vi "Ex 06 - B-Scan.vi"() -> ()   [LabVIEW 2026]
uses:
  <instrlib>/MicroPulse/Public/Data/Datatypes/MP - data formatting.ctl
  <instrlib>/MicroPulse/Public/Data/Datatypes/MP - amplitude reporting mode.ctl
  <instrlib>/MicroPulse/Public/Data/Datatypes/MP - averaging.ctl
  <instrlib>/MicroPulse/Public/Data/Datatypes/MP - transmit parameters.ctl
  <instrlib>/MicroPulse/Public/Data/Datatypes/MP - pulser voltage.ctl
  <instrlib>/MicroPulse/Public/Data/Datatypes/MP - pulse damping.ctl
  <instrlib>/MicroPulse/Public/Data/Datatypes/MP - test parameters.ctl
  <instrlib>/MicroPulse/Public/Data/Datatypes/MP - receive parameters.ctl
  <instrlib>/MicroPulse/Public/Data/Datatypes/MP - display gate.ctl
  <instrlib>/MicroPulse/Public/Data/Datatypes/MP - waveform type.ctl
  <instrlib>/MicroPulse/Public/Data/Datatypes/MP - analogue filter.ctl
  <instrlib>/MicroPulse/Public/Data/Datatypes/MP - frequency filter.ctl
  <instrlib>/MicroPulse/Public/Data/Datatypes/MP - digital filtering.ctl
  <instrlib>/MicroPulse/Public/Data/Datatypes/MP - high pass filter.ctl
  <instrlib>/MicroPulse/Public/Data/Datatypes/MP - low pass filter.ctl
  <instrlib>/MicroPulse/Public/Data/Datatypes/TCP config.ctl
  <instrlib>/MicroPulse/Public/Data/Datatypes/MP - multi-gate inspection.ctl
  <instrlib>/MicroPulse/Public/Data/Datatypes/MP - multigate inspection gate parameters.ctl
  <instrlib>/MicroPulse/Public/Data/Datatypes/MP - hysteresis level.ctl
  <instrlib>/MicroPulse/Public/Data/Datatypes/MP - multigate mode.ctl
  <instrlib>/MicroPulse/Public/Data/Datatypes/MP - echo gate parameters.ctl
  <instrlib>/MicroPulse/Public/Data/Datatypes/MP - echo gate mode.ctl
  <instrlib>/MicroPulse/Public/Data/Datatypes/MP - data output format.ctl
  <instrlib>/MicroPulse/Public/Data/Datatypes/MP - sample frequency.ctl
  <instrlib>/MicroPulse/Public/Data/Datatypes/MP - instrument type.ctl
  <instrlib>/MicroPulse/Public/Data/Datatypes/MP - fly scan range.ctl
  <instrlib>/MicroPulse/Public/Data/Datatypes/MP - inspection direction.ctl
  <instrlib>/MicroPulse/Public/Data/Datatypes/MP - encoder settings.ctl
  <instrlib>/MicroPulse/Public/Data/Datatypes/MP - encoder type.ctl
  <instrlib>/MicroPulse/Public/Data/Datatypes/MP - request system status.ctl
  <instrlib>/MicroPulse/Public/Data/Datatypes/MP - encoder mode.ctl
  <instrlib>/MicroPulse/Public/Data/Datatypes/MP - fly scan range (relative).ctl
  <instrlib>/MicroPulse/Public/Data/Datatypes/MP - inspection direction (relative).ctl
  <instrlib>/MicroPulse/Public/Data/Datatypes/MP - fly scan range (timed).ctl
  <instrlib>/MicroPulse/Public/Data/Datatypes/PNDT - colour map selector.ctl
  <instrlib>/MicroPulse/Examples/SubVIs/Main Program State - Enum.ctl
  <instrlib>/MicroPulse/Public/Data/Datatypes/MP - fly inspection tests.ctl
  <instrlib>/MicroPulse/Public/Helper VIs/Low Level/FGV - B-Scan Active - Action [Enum].ctl
  <vilib>/ErrorRing/Error Ring.xnode
  <instrlib>/MicroPulse/MicroPulse_Driver.lvlib
panel:
  in  "Centre Cursor":bool
  in  "Get Status":bool
  in  "Colour Map":T1
  out "B-Scan In Progress?":bool
  in  "Stop Test":bool
  out "B-Scan Chart":u16[][](graph)
  in  "Request System Status":T2 caption="[STS]"
  out "Current Position":dbl format="%#_6f mm"
  in  "Test Tab":T3(tab)
  in  "Data Formatting":T4={"Amplitude Mode"=enum."Peaks + Ascan for Multigate", "Averaging"=enum."None", "Coupling Level"=0} {"Coupling Level" max=4095 step=1}
  in  "Transmit Parameters":T7={"Pulse Voltage"=enum."50V", "Pulse Shape"={"Damping"=enum."660W", "Width"=250}} {"Pulse Shape"."Width" min=16 max=1010 step=50 format="%.0fns"}
  in  "Test Parameters":T10={"Test No."=1, "Tx Channel"=1, "Rx Channel"=1} {"Rx Channel" min=1 max=1024; "Tx Channel" min=1 max=1024}
  in  "Receive Parameters":T11={"Display Gate"={"Start"=0.0, "Length"=100.0}, "Delay"=0.0, "Waveform Type"=enum."Rectified Signal", "Gain"=50.0, "Analogue Filtering"={"Bandpass"=enum."No change", "Smoothing"=1}, "Digital Filtering"={"High Pass Filter"=enum."None", "Low Pass Filter"=enum."None"}} {"Delay" format="%#_g us"; "Display Gate"."Length" min=0.0 max=64000.0 step=1.0 format="%#_g us"; "Display Gate"."Start" min=0.0 max=64000.0 step=1.0 format="%#_g us"; "Analogue Filtering"."Smoothing" min=1 max=11 step=1; "Gain" min=-6.0 max=70.0 step=0.25 format="%.2fdB"}
  in  "Multi Gate Inspection":T19={"Gate 1"={"Start (us)"=15.0, "Length (us)"=10.0, "Threshold"=80, "Enabled?"=TRUE, "Max # Peaks"=8, "Hysteresis"=enum."6dB", "Mode"=enum."All Peaks In Gate", "Inverted?"=FALSE, "Colour "=16716306}, "Gate 2"={"Start (us)"=30.0, "Length (us)"=10.0, "Threshold"=50, "Enabled?"=TRUE, "Max # Peaks"=8, "Hysteresis"=enum."6dB", "Mode"=enum."All Peaks In Gate", "Inverted?"=FALSE, "Colour "=641024}, "Gate 3"={"Start (us)"=50.0, "Length (us)"=10.0, "Threshold"=30, "Enabled?"=TRUE, "Max # Peaks"=8, "Hysteresis"=enum."6dB", "Mode"=enum."All Peaks In Gate", "Inverted?"=FALSE, "Colour "=4532}, "Gate 4"={"Start (us)"=65.0, "Length (us)"=10.0, "Threshold"=10, "Enabled?"=TRUE, "Max # Peaks"=8, "Hysteresis"=enum."6dB", "Mode"=enum."All Peaks In Gate", "Inverted?"=FALSE, "Colour "=8978537}} {"Gate 4"."Max # Peaks" min=1 max=80 step=1; "Gate 4"."Threshold" min=10 step=10; "Gate 4"."Length (us)" min=0.0 max=96000.0 step=1.0; "Gate 4"."Start (us)" min=0.0 max=64000.0 step=1.0; "Gate 3"."Max # Peaks" min=1 max=80 step=1; "Gate 3"."Threshold" min=10 step=10; "Gate 3"."Length (us)" min=0.0 max=96000.0 step=1.0; "Gate 3"."Start (us)" min=0.0 max=64000.0 step=1.0; "Gate 2"."Max # Peaks" min=1 max=80 step=1; "Gate 2"."Threshold" min=10 step=10; "Gate 2"."Length (us)" min=0.0 max=96000.0 step=1.0; "Gate 2"."Start (us)" min=0.0 max=64000.0 step=1.0; "Gate 1"."Max # Peaks" min=1 max=80 step=1; "Gate 1"."Threshold" min=10 step=10; "Gate 1"."Length (us)" min=0.0 max=96000.0 step=1.0; "Gate 1"."Start (us)" min=0.0 max=64000.0 step=1.0}
  in  "Echo Gate Parameters":T23={"Start (us)"=15.0, "Length (us)"=20.0, "Threshold"=10, "Colour"=2731480} {"Threshold" min=10 max=4095 step=10; "Length (us)" min=0.0 max=96000.0 step=1.0; "Start (us)" min=0.0 max=64000.0 step=1.0}
  in  "Echo Gate Mode":T24
  in  "Encoder Reporting Mode":T25=enum."32-bit + LLC" caption="[ENCM]"
  in  "Set Position":bool
  in  "Position To Set":dbl caption="mm"
  in  "Encoder Settings":T26={"Encoder Type"=enum."Quadrature", "Counts/mm"=100, "Enable Termination?"=FALSE, "Multiplier"=2, "Backlash Period (s)"=10.0, "Encoder Filter"=0} {"Encoder Filter" max=255; "Backlash Period (s)" min=0.0005 max=10.0 step=0.0005; "Multiplier" min=1 max=100000; "Counts/mm" min=1 max=100000}
  in  "Axis No.":u8=1 min=1 max=4
  in  "Scan Choice":T28(tab)
  in  "FLZ Scan definition":T29={"Scan Start"=0.0, "Scan Length"=280.0, "Inspection Resolution"=0.5, "Direction"=enum."Forwards"} {"Inspection Resolution" format="%#_6f"; "Scan Start" format="%#_6f"; "Scan Length" format="%#_6f"}
  in  "Start FLZ Test":bool
  in  "FLR Scan definition":T31={"Scan Length"=0.0, "Inspection Resolution"=1.0, "Direction"=enum."Bidirectional"} {"Inspection Resolution" format="%#_6f"; "Scan Length" format="%#_6f"}
  in  "Start FLR Test":bool
  out "Scan Timer Enabled?":bool
  in  "Start Timed Test":bool
  in  "Timed Scan definition":T33={"Max Scan Length"=0, "Update Rate"=1000, "Direction"=enum."Forwards"} {"Update Rate" format="%#_6f"; "Max Scan Length" format="%#_6f"}
  out "Instrument Type":T34
  out "Sample Frequency out":T35 caption="Sample Frequency"
  out "Stop":bool
  in  "Sample Frequency":T35
  in  "PRF":u16=20000 caption="[PRF]" min=1 max=20000 step=100 format="%dHz"
  in  "Data Output Format":T36=enum."8-bit Mode" caption="[DOF]"
  in  "Gate No.":i32=1
  out "peak data":cluster{"Time":dbl[], "Level":u16[]} {"Time" format="%_6g"}
  out "A-Scan + Peaks":cluster{"timebase":dbl[], "data":u16[]}[](graph) caption="A-Scan + Peaks Test 1"
  in  "Acquire Single Scan":bool
  in  "Stop Acquisition":bool
  in  "Start Acquisition":bool
  out "Command List":string
  in  "QUIT":bool
  out "running average PRF":dbl format="%0.2f"
  out "live error out":errorcluster
  out "message count":i32
  out "System Messages":string
  in  "TCP config":T37={"Connection ID"=refnum, "IP address"="10.1.1.2", "host port"=1067, "OC timeout"=5000, "Read timeout"=2000, "Write timeout"=100} {"Write timeout" format="%dms"; "Read timeout" format="%dms"; "OC timeout" format="%dms"}
  # "Example 06 - B-Scans\n\nSet all controls to the required values\nbefore running the VI.\n\nWhile running, test parameters may NOT be  changed."
  # "Multiplier of 2 sets the inspection resolution to 1/2 of the base unit.\nBase unit is set by  \"Counts/mm\""
  # "Set Current Position"
  # "Set to zero for unlimited points. Requires manual stop."
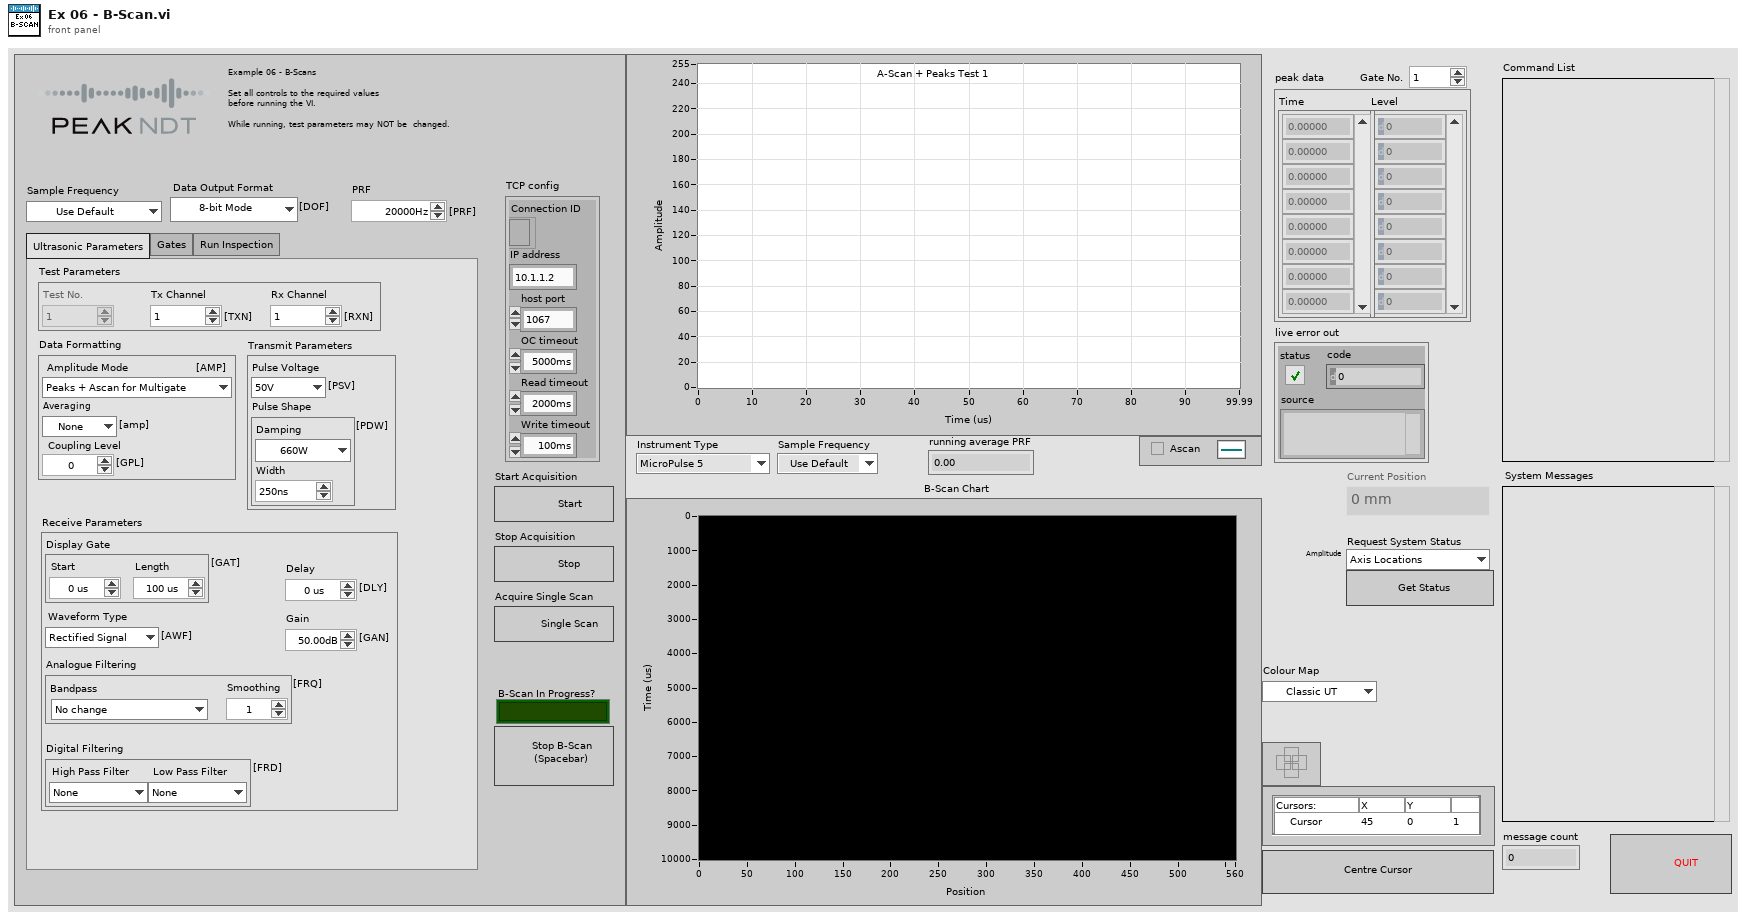
[diagram p1: front panel]
types:
  T1 = typedef "MicroPulse_Driver.lvlib/PNDT - colour map selector.ctl" = enum16{"Classic UT", "Ultrasonic", "Inverse Grey", "Grey Scale", "TOFD", "Fire", "Rainbow", "Ice", "Original"}
  T2 = typedef "MicroPulse_Driver.lvlib/MP - request system status.ctl" = enum16{"Axis Locations", "MPE settings", "BKL settings", "SPA settings", "I/O status", "RST elapsed time", "System Status", "Temperatures", "System Log", "Erase system Log", "RST message", "Master System Msg", "Slave System Msg"}
  T3 = enum32{"Ultrasonic Parameters", "Gates", "Run Inspection"}
  T4 = typedef "MicroPulse_Driver.lvlib/MP - data formatting.ctl" = cluster{"Amplitude Mode":T5, "Averaging":T6, "Coupling Level":u32}
  T5 = typedef "MicroPulse_Driver.lvlib/MP - amplitude reporting mode.ctl" = enum16{"1st Peak in gate", "Maximum Peak in gate", "All Peaks", "Ascan Data", "1st Threshold Crossing Peak", "Ascan + Peaks", "All Peaks for Multigate", "Peaks + Ascan for Multigate", "Peaks + P_Ascan for Multigate", "Full Matrix Capture"}
  T6 = typedef "MicroPulse_Driver.lvlib/MP - averaging.ctl" = enum16{"None", "2", "4", "8", "16", "32", "64", "128", "256"}
  T7 = typedef "MicroPulse_Driver.lvlib/MP - transmit parameters.ctl" = cluster{"Pulse Voltage":T8, "Pulse Shape":cluster{"Damping":T9, "Width":u32}}
  T8 = typedef "MicroPulse_Driver.lvlib/MP - pulser voltage.ctl" = enum16{"50V", "100V", "150V", "200V", "250V", "300V"}
  T9 = typedef "MicroPulse_Driver.lvlib/MP - pulse damping.ctl" = enum16{"660W", "458W", "220W", "149W", "102W", "82W", "63W", "51W"}
  T10 = typedef "MicroPulse_Driver.lvlib/MP - test parameters.ctl" = cluster{"Test No.":u32, "Tx Channel":u32, "Rx Channel":u32}
  T11 = typedef "MicroPulse_Driver.lvlib/MP - receive parameters.ctl" = cluster{"Display Gate":T12, "Delay":dbl, "Waveform Type":T13, "Gain":dbl, "Analogue Filtering":T14, "Digital Filtering":T16}
  T12 = typedef "MicroPulse_Driver.lvlib/MP - display gate.ctl" = cluster{"Start":dbl, "Length":dbl}
  T13 = typedef "MicroPulse_Driver.lvlib/MP - waveform type.ctl" = enum16{"Rectified Signal", "RF Signal", "+Half Wave", "-Half Wave"}
  T14 = typedef "MicroPulse_Driver.lvlib/MP - analogue filter.ctl" = cluster{"Bandpass":T15, "Smoothing":u16}
  T15 = typedef "MicroPulse_Driver.lvlib/MP - frequency filter.ctl" = enum16{"No change", "1MHz Bandpass", "2MHz Bandpass", "4MHz Bandpass", "5MHz Bandpass", "10MHz Bandpass", "2.5-18MHz Broadband", "0.75-12MHz  Broadband", "0.5MHz Bandpass", "5MHz 2nd Order TOFD", "10MHz 2nd Order TOFD", "3.0-25MHz Broadband", "3.0-30MHz Broadband"}
  T16 = typedef "MicroPulse_Driver.lvlib/MP - digital filtering.ctl" = cluster{"High Pass Filter":T17, "Low Pass Filter":T18}
  T17 = typedef "MicroPulse_Driver.lvlib/MP - high pass filter.ctl" = enum16{"None", "0.7MHz", "1.5MHz", "4.0MHz", "7.5MHz", "10.0MHz", "User Defined"}
  T18 = typedef "MicroPulse_Driver.lvlib/MP - low pass filter.ctl" = enum16{"None", "1.8MHz", "3.0MHz", "6.0MHz", "8.0MHz", "12.0MHz", "User Defined"}
  T19 = typedef "MicroPulse_Driver.lvlib/MP - multi-gate inspection.ctl" = cluster{"Gate 1":T20, "Gate 2":T20, "Gate 3":T20, "Gate 4":T20}
  T20 = typedef "MicroPulse_Driver.lvlib/MP - multigate inspection gate parameters.ctl" = cluster{"Start (us)":dbl, "Length (us)":dbl, "Threshold":u16, "Enabled?":bool, "Max # Peaks":u16, "Hysteresis":T21, "Mode":T22, "Inverted?":bool, "Colour ":u32}
  T21 = typedef "MicroPulse_Driver.lvlib/MP - hysteresis level.ctl" = enum16{"None", "3dB", "6dB", "9dB", "12dB"}
  T22 = typedef "MicroPulse_Driver.lvlib/MP - multigate mode.ctl" = enum16{"1st Peak in Gate", "Largest Peak In Gate", "All Peaks In Gate", "1st Threshold Crossing"}
  T23 = typedef "MicroPulse_Driver.lvlib/MP - echo gate parameters.ctl" = cluster{"Start (us)":dbl, "Length (us)":dbl, "Threshold":u16, "Colour":u32}
  T24 = typedef "MicroPulse_Driver.lvlib/MP - echo gate mode.ctl" = enum16{"Echo Trigger OFF", "Echo Gate Display Mode", "Echo Trigger ON", "Multi Gate or FMC Mode", "Reserved", "PA - Echo Trigger ON"}
  T25 = typedef "MicroPulse_Driver.lvlib/MP - encoder mode.ctl" = enum16{"24-bit + LCI", "32-bit + LCI", "32-bit + LLC", "24-bit + STS6", "32-bit + STS6", "32-bit + LLC+STS6"}
  T26 = typedef "MicroPulse_Driver.lvlib/MP - encoder settings.ctl" = cluster{"Encoder Type":T27, "Counts/mm":u32, "Enable Termination?":bool, "Multiplier":u32, "Backlash Period (s)":dbl, "Encoder Filter":u32}
  T27 = typedef "MicroPulse_Driver.lvlib/MP - encoder type.ctl" = enum16{"Quadrature", "Step/Direction"}
  T28 = enum32{"Absolute Scan [FLX+FLZ]", "Relative Scan [FLR] ", "Timed Scan"}
  T29 = typedef "MicroPulse_Driver.lvlib/MP - fly scan range.ctl" = cluster{"Scan Start":dbl, "Scan Length":dbl, "Inspection Resolution":dbl, "Direction":T30}
  T30 = typedef "MicroPulse_Driver.lvlib/MP - inspection direction.ctl" = enum16{"Forwards", "Backwards"}
  T31 = typedef "MicroPulse_Driver.lvlib/MP - fly scan range (relative).ctl" = cluster{"Scan Length":dbl, "Inspection Resolution":dbl, "Direction":T32}
  T32 = typedef "MicroPulse_Driver.lvlib/MP - inspection direction (relative).ctl" = enum16{"Forwards", "Backwards", "Bidirectional"}
  T33 = typedef "MicroPulse_Driver.lvlib/MP - fly scan range (timed).ctl" = cluster{"Max Scan Length":i32, "Update Rate":i32, "Direction":T30}
  T34 = typedef "MicroPulse_Driver.lvlib/MP - instrument type.ctl" = enum16{"MicroPulse 5", "LT1", "LT2", "LTPA", "MPLT", "MicroPulse 6", "PipeScanner", "<MicroPulse>", "Micropulse 4", "Simulated Data"}
  T35 = typedef "MicroPulse_Driver.lvlib/MP - sample frequency.ctl" = enum16{"Use Default", "200MHz (LT2 only)", "100MHz", "50MHz", "25MHz", "10MHz"}
  T36 = typedef "MicroPulse_Driver.lvlib/MP - data output format.ctl" = enum16{"", "8-bit Mode", "10-bit Mode", "12-bit Mode", "16-bit Mode", "8-bit Log Mode", "12-bit Packed Mode"}
  T37 = typedef "MicroPulse_Driver.lvlib/TCP config.ctl" = cluster{"Connection ID":refnum<k5>, "IP address":string, "host port":u16, "OC timeout":i32, "Read timeout":i32, "Write timeout":i32}
  T38 = typedef "Main Program State - Enum.ctl" = enum16{"Initialise", "Init HW", "Run", "Reset HW", "Shutdown"}
  T39 = typedef "MicroPulse_Driver.lvlib/FGV - B-Scan Active - Action [Enum].ctl" = enum16{"Read", "Read & Reset Start Flag", "Start B-Scan", "B-Scan Finished"}
  T40 = typedef "MicroPulse_Driver.lvlib/MP - fly inspection tests.ctl" = enum16{"Conventional Tests", "Conv >> PA Tests", "PA >> Conv Tests", "PA Tests", "Group Tests", "PA Sweep as per FDEF"}
  T41 = typedef "MicroPulse_Driver.lvlib/MP-Registry Data-Cluster.ctl" = cluster{"Instrument Type":T34, "Serial #":u64, "Sample Frequency":T35, "dt (us)":dbl, "DOF":T36, "Material Velocity":dbl, "Asynch Reads":T42, "NUM of Tests":u32, "System Details":T43, "Gates":T45[], "Encoders":T26[], "CMD LUT":variant, "Command List":string}
  T42 = typedef "MicroPulse_Driver.lvlib/MP - asynch read mode.ctl" = enum16{"Disabled", "Enabled"}
  T43 = typedef "MicroPulse_Driver.lvlib/MP - general system status.ctl" = cluster{"System Type":T34, "Serial No.":u64, "Channels":cluster{"Conv":u8, "PA":u16, "Extra":u32}, "Sample Frequency":cluster{"Default":u8, "Actual":u8}, "Software Versions":string, "Data Output Format":cluster{"Default":T36, "Actual":T36}, "Temperatures":cluster{"System":u8, "Processor":u8, "Slave Sys":u8, "Slave Proc":u8}, "Tx Buffer Size":u32, "System Error":string, "No. of Cards":u8, "DAC Gain":i16, "Uptimes":cluster{"since Power":u32, "since RSTS":u32, "since SRST":u32}, "Voltages":cluster{"Nominal":dbl, "Measured":dbl, "Difference":dbl}[], "Interface Cards":T44[]}
  T44 = typedef "MicroPulse_Driver.lvlib/MP - interface card status.ctl" = cluster{"Status":u8, "Map":u8, "Board - T":u8, "FPGA - T":u8, "PAIF Status":string, "Version":string}
  T45 = typedef "MicroPulse_Driver.lvlib/MP - Registry Gates.ctl" = cluster{"Display Gate":T12, "ETM Mode":T24, "Echo Gate":T23, "Insp Gates":T20[]}
  T46 = typedef "LVPointDoubleTypeDef.ctl" = cluster{"Cursor X":dbl, "Cursor Y":dbl}
  T47 = typedef "LVBoundsTypeDef.ctl" = cluster{"Width":u32, "Height":u32}
  T48 = typedef "MicroPulse_Driver.lvlib/MP - scan data info.ctl" = cluster{"Message Header":u16, "Error Message":u16, "Test No.":u32, "Channel No.":u8, "Sweep No.":u32, "Gate No.":u32, "DOF":T36, "retain data":T49, "scan data":u16[], "scan length":i32, "scan index":i32, "peak data":cluster{"timebase":u16[], "data":u16[]}, "#peaks":i32, "PRF":dbl, "IP":cluster{"Axis No.":u8, "Location":u32, "MIP location":u32, "MIP?":bool}, "echo range":u16, "ETG":bool, "CAL 0 complete":bool, "Axis Positions":T50}
  T49 = typedef "MicroPulse_Driver.lvlib/MP - retain scan.ctl" = enum16{"None", "Ascan", "Peaks"}
  T50 = typedef "MicroPulse_Driver.lvlib/MP - axis positions (LLC).ctl" = cluster{"Axis 1":u32, "Axis 2":u32, "Axis 3":u32, "Axis 4":u32, "Status":u8}
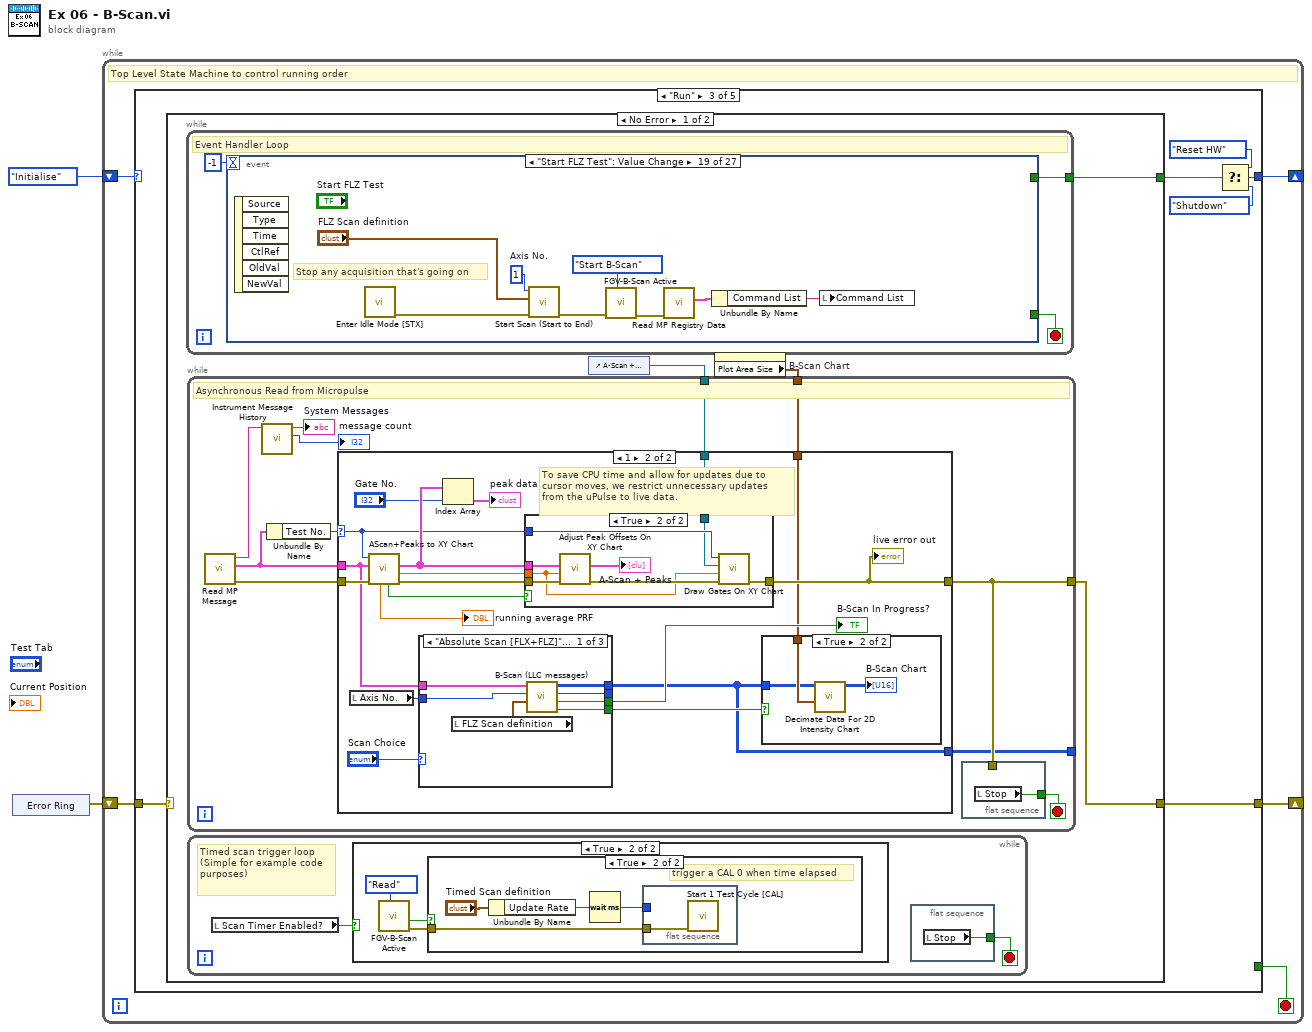
[diagram p0: block diagram]
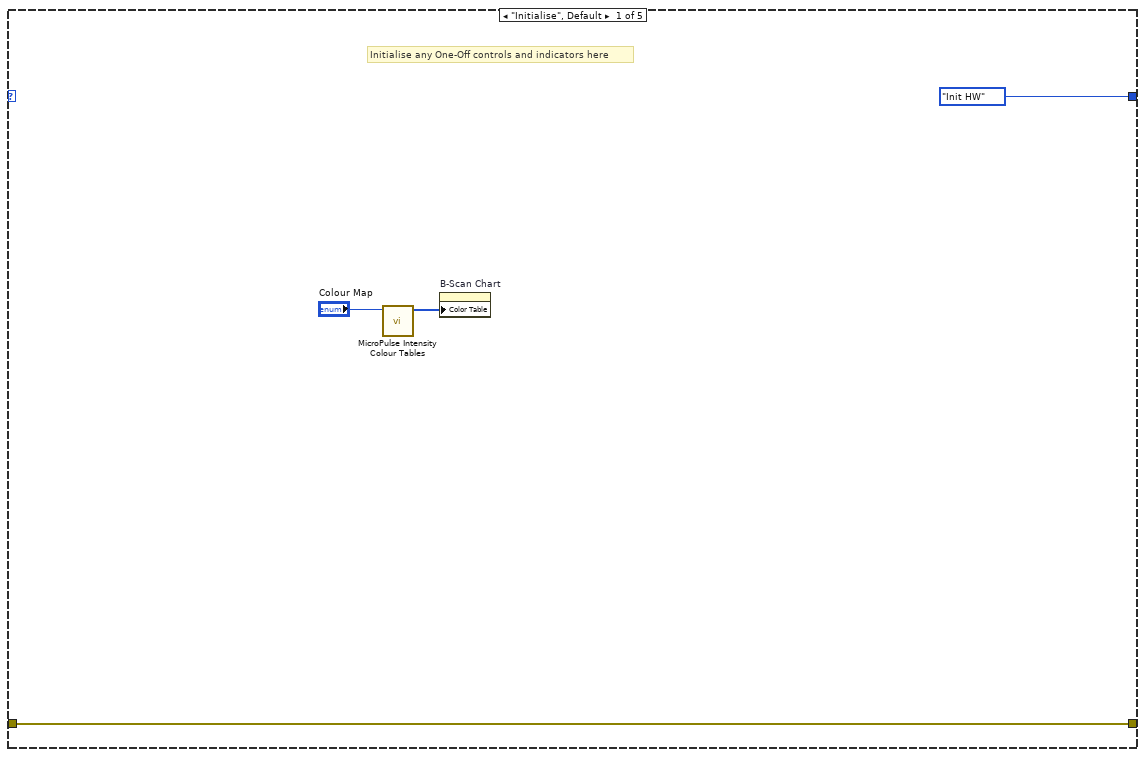
[diagram p2: hidden frame]
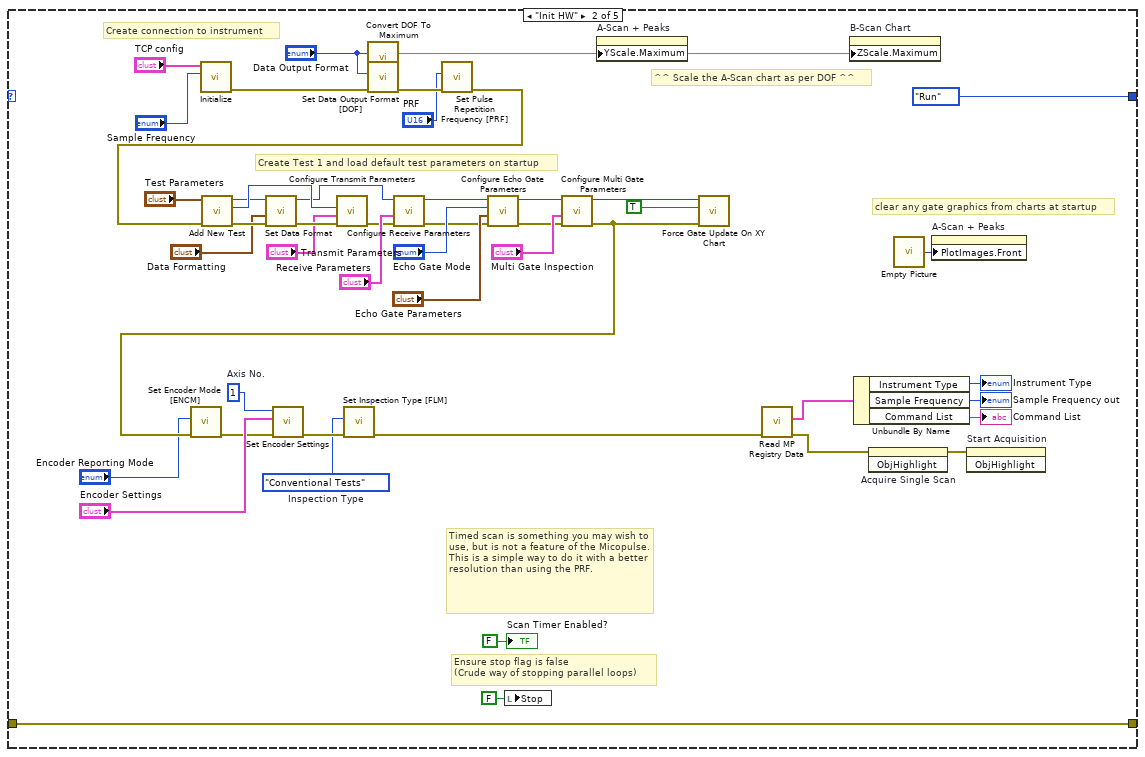
[diagram p3: hidden frame]
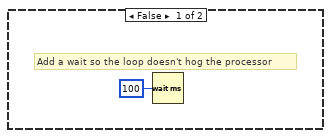
[diagram p4: hidden frame]
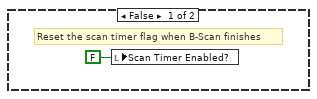
[diagram p5: hidden frame]
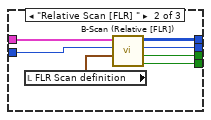
[diagram p9: hidden frame]
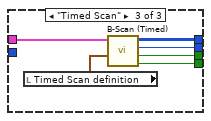
[diagram p10: hidden frame]
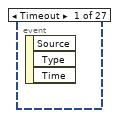
[diagram p11: hidden frame]
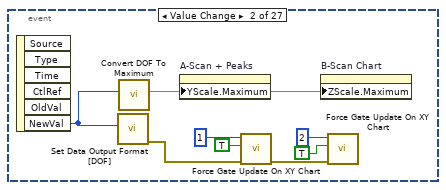
[diagram p12: hidden frame]
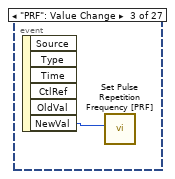
[diagram p13: hidden frame]
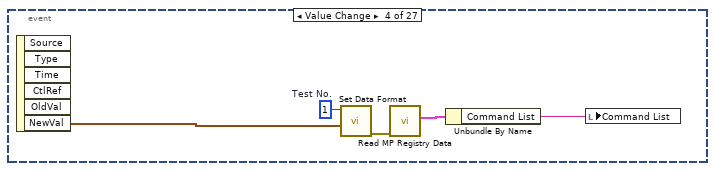
[diagram p14: hidden frame]
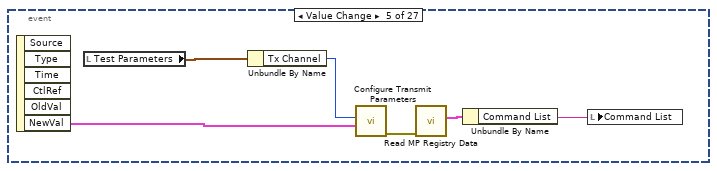
[diagram p15: hidden frame]
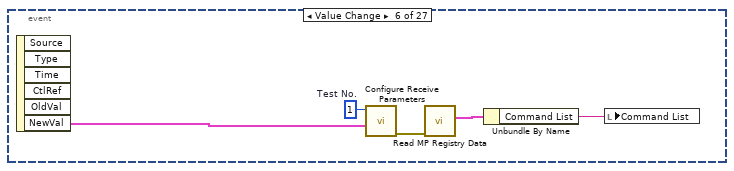
[diagram p16: hidden frame]
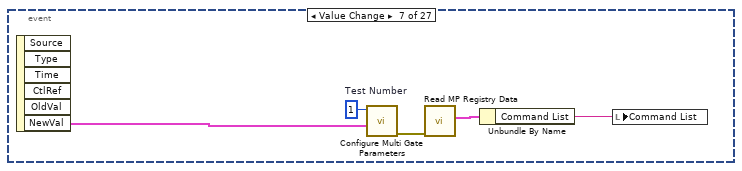
[diagram p17: hidden frame]
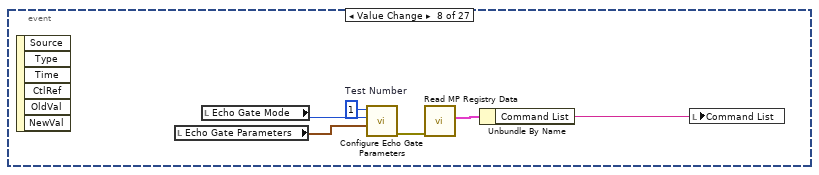
[diagram p18: hidden frame]
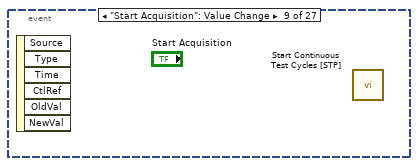
[diagram p19: hidden frame]
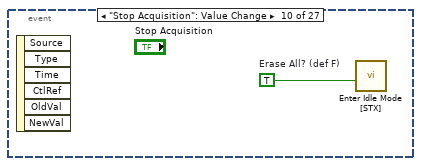
[diagram p20: hidden frame]
diagram:
  n1 = xnode "Error Ring"() -> ("error out"=w2:errorcluster)
  n2 = while {
    shift-right: [w4] -> _
    shift-left: Main_Program_State_-_Enum."Initialise" -> [w7]
    shift-right: [w5] -> _
    shift-left: w2 -> [w6]
    stop <- w3 stop-if-true
    # "Top Level State Machine to control running order"
    n3 = case shown="\"Run\"" w7 {
      tunnel: w6 -> [w10 w35 w63 w252 w257]
      tunnel: [w10 w35 w62 w251 w257] -> w5
      tunnel: [Main_Program_State_-_Enum."Init HW" Main_Program_State_-_Enum."Run" w58 Main_Program_State_-_Enum."Init HW" Main_Program_State_-_Enum."Initialise"] -> w4
      tunnel: [_ _ _ _ TRUE] -> w3
      frame "Initialise", Default {
        # "Initialise any One-Off controls and indicators here"
        n4 = call <instrlib>:"MicroPulse Intensity Colour Tables.vi"("Colour Map Type"="Colour Map") -> ("Colour Table"=w8:u32[])  [unwired: 10 in]
        n5 = property on="B-Scan Chart" class="IntGraph (strict)"("Color Table"=w8) -> ()  [unwired: 2 in, 2 out]
      }
      frame "Init HW" {
        w14 = MP_-_fly_inspection_tests."Conventional Tests"  # Inspection Type
        w17 = u8 1  # Axis No.
        # "Timed scan is something you may wish to use, but is not a feature of the Micopulse.\nThis is a simple way to do it with a better resolution than using the PRF."
        # "^^ Scale the A-Scan chart as per DOF ^^"
        # "Ensure stop flag is false\n(Crude way of stopping parallel loops)"
        # "Create connection to instrument"
        # "clear any gate graphics from charts at startup"
        # "Create Test 1 and load default test parameters on startup"
        n6 = call <instrlib>:"Initialize.vi"("Sample Frequency"="Sample Frequency", "TCP config"="TCP config") -> ("error out"=w26:errorcluster)  [unwired: 8 in, 1 out]
        n7 = call <instrlib>:"Convert DOF To Maximum.vi"("Data Output Format"="Data Output Format") -> ("Data Maximum"=w13:dbl)  [unwired: 10 in]
        n8 = call <instrlib>:"Set Data Output Format [DOF].vi"("error in (no error)"=w26, "Mode"="Data Output Format") -> ("error out"=w28:errorcluster)  [unwired: 8 in, 1 out]
        n9 = call <instrlib>:"Set Pulse Repetition Frequency [PRF].vi"("error in (no error)"=w28, "Frequency (Hz)"="PRF") -> ("error out"=w25:errorcluster)  [unwired: 8 in, 1 out]
        n10 = call <instrlib>:"Add New Test.vi"("error in (no error)"=w25, "Test Parameters"="Test Parameters") -> ("error out"=w50:errorcluster, "Tx Channel out"=w49:u32, "Test No. out"=w45:u32)  [unwired: 6 in, 1 out]
        n11 = call <instrlib>:"Set Data Format.vi"("error in (no error)"=w50, "Data Formatting"="Data Formatting", "Test No."=w45) -> ("error out"=w40:errorcluster, "Test No. out"=w47:u32)  [unwired: 6 in, 1 out]
        n12 = call <instrlib>:"Configure Transmit Parameters.vi"("error in (no error)"=w40, "Transmit Parameters"="Transmit Parameters", "Tx Channel"=w49) -> ("error out"=w39:errorcluster)  [unwired: 7 in, 1 out]
        n13 = call <instrlib>:"Configure Receive Parameters.vi"("error in (no error)"=w39, "Receive Parameters"="Receive Parameters", "Test No."=w47) -> ("error out"=w41:errorcluster, "Test No. out"=w46:u32)  [unwired: 6 in, 1 out]
        n14 = call <instrlib>:"Configure Echo Gate Parameters.vi"("error in (no error)"=w41, "Echo Gate Parameters"="Echo Gate Parameters", "Echo Trigger Mode"="Echo Gate Mode", "Test Number"=w46) -> ("error out"=w43:errorcluster, "Test Number Out"=w48:u32)  [unwired: 5 in, 1 out]
        n15 = local write "Stop"(FALSE ("stop")) -> ()
        n16 = call <instrlib>:"Configure Multi Gate Parameters.vi"("error in (no error)"=w43, "Multi Gate Inspection"="Multi Gate Inspection", "Test Number"=w48) -> ("error out"=w21:errorcluster, "Test Number out"=w33:u32)  [unwired: 6 in, 1 out]
        n17 = call <instrlib>:"Set Encoder Mode [ENCM].vi"("error in (no error)"=w21, "Encoder Mode"="Encoder Reporting Mode") -> ("error out"=w18:errorcluster)  [unwired: 8 in, 1 out]
        n18 = call <instrlib>:"Set Encoder Settings.vi"("error in (no error)"=w18, "Encoder Settings"="Encoder Settings", "Axis No."=w17) -> ("error out"=w16:errorcluster)  [unwired: 8 in]
        n19 = call <instrlib>:"Set Inspection Type [FLM].vi"("error in (no error)"=w16, "Inspection Type"=w14) -> ("error out"=w15:errorcluster)  [unwired: 8 in, 1 out]
        n20 = property on="A-Scan + Peaks" class="XYGraph (strict)"("YScale.Maximum"=w13) -> ()  [unwired: 2 in, 2 out]
        n21 = call <instrlib>:"Force Gate Update On XY Chart.vi"("error in (no error)"=w21, "Set?"=TRUE, "Test No."=w33) -> ()  [unwired: 6 in, 3 out]
        n22 = call <instrlib>:"Read MP Registry Data.vi"("error in (no error)"=w15) -> ("error out"=w56:errorcluster, "Micropulse Data"=w54:T41)  [unwired: 7 in, 2 out]
        n23 = property on="B-Scan Chart" class="IntGraph (strict)"("ZScale.Maximum"=w13) -> ()  [unwired: 2 in, 2 out]
        n24 = Unbundle By Name(w54) -> ("Instrument Type"=→"Instrument Type":T34, "Sample Frequency"=→"Sample Frequency out":T35, "Command List"=→"Command List":string)
        n25 = invoke on="Acquire Single Scan" class="Bool" method="ObjHighlight"(error in=w56) -> (error out=w57:errorcluster)  [unwired: 2 in, 2 out]
        n26 = call "Empty Picture"() -> ("empty picture"=w34:picture)
        n27 = property on="A-Scan + Peaks" class="XYGraph (strict)"("PlotImages.Front"=w34) -> ()  [unwired: 2 in, 2 out]
        n28 = invoke on="Start Acquisition" class="Bool" method="ObjHighlight"(error in=w57) -> ()  [unwired: 2 in, 3 out]
        "Scan Timer Enabled?" <- FALSE ("Scan Timer Enabled?")
      }
      frame "Run" {
        n29 = case shown="No Error" w63 {
          selector: w63 -> [_ w250]
          tunnel: [w64 w250] -> w62
          tunnel: [w66 FALSE] -> w59
          frame No Error {
            n30 = while {
              tunnel: [w145] -> w66
              stop <- w146 stop-if-true
              # "Event Handler Loop"
              n31 = event shown="[18] \"Start FLZ Test\": Value Change" {
                selector: _ -> [_ _ _ _ _ _ _ _ _ _ _ _ _ _ _ _ _ _ _ _ _ _ _ _ _ _ _]
                dyn-events: _ -> [_ _ _ _ _ _ _ _ _ _ _ _ _ _ _ _ _ _ _ _ _ _ _ _ _ _ _]
                timeout: -1 -> [_ _ _ _ _ _ _ _ _ _ _ _ _ _ _ _ _ _ _ _ _ _ _ _ _ _ _]
                tunnel: [_ _ _ _ _ _ _ _ _ _ _ _ w186 _ _ _ _ _ _ _ _ _ _ _ _ _ TRUE ("stop")] -> w146
                tunnel: [_ _ _ _ _ _ _ _ _ _ _ _ TRUE _ _ _ _ _ _ _ _ _ _ _ _ FALSE _] -> w145
                event Timeout {
                  n32 = event-data() -> ()  [unwired: 1 in, 3 out]
                }
                event Value Change {
                  n33 = event-data() -> ("NewVal"=w148:T36)  [unwired: 1 in, 5 out]
                  n34 = call <instrlib>:"Set Data Output Format [DOF].vi"("Mode"=w148) -> ("error out"=w150:errorcluster)  [unwired: 9 in, 1 out]
                  n35 = call <instrlib>:"Convert DOF To Maximum.vi"("Data Output Format"=w148) -> ("Data Maximum"=w147:dbl)  [unwired: 10 in]
                  n36 = property on="A-Scan + Peaks" class="XYGraph (strict)"("YScale.Maximum"=w147) -> ()  [unwired: 2 in, 2 out]
                  n37 = call <instrlib>:"Force Gate Update On XY Chart.vi"("error in (no error)"=w150, "Set?"=TRUE, "Test No."=u32 1) -> ("error out"=w149:errorcluster)  [unwired: 6 in, 2 out]
                  n38 = property on="B-Scan Chart" class="IntGraph (strict)"("ZScale.Maximum"=w147) -> ()  [unwired: 2 in, 2 out]
                  n39 = call <instrlib>:"Force Gate Update On XY Chart.vi"("error in (no error)"=w149, "Set?"=TRUE, "Test No."=u32 2) -> ()  [unwired: 6 in, 3 out]
                }
                event "PRF": Value Change {
                  n40 = event-data() -> ("NewVal"=w155:u16)  [unwired: 1 in, 5 out]
                  n41 = call <instrlib>:"Set Pulse Repetition Frequency [PRF].vi"("Frequency (Hz)"=w155) -> ()  [unwired: 9 in, 2 out]
                }
                event Value Change {
                  w157 = u32 1  # Test No.
                  n42 = event-data() -> ("NewVal"=w156:T4)  [unwired: 1 in, 5 out]
                  n43 = call <instrlib>:"Set Data Format.vi"("Data Formatting"=w156, "Test No."=w157) -> ("error out"=w160:errorcluster)  [unwired: 7 in, 2 out]
                  n44 = call <instrlib>:"Read MP Registry Data.vi"("error in (no error)"=w160) -> ("Micropulse Data"=w159:T41)  [unwired: 7 in, 3 out]
                  n45 = Unbundle By Name(w159) -> ("Command List"=w158:string)
                  n46 = local write "Command List"(w158) -> ()
                }
                event Value Change {
                  n47 = event-data() -> ("NewVal"=w165:T7)  [unwired: 1 in, 5 out]
                  n48 = local read "Test Parameters"() -> (w166:T10)
                  n49 = Unbundle By Name(w166) -> ("Tx Channel"=w164:u32)
                  n50 = call <instrlib>:"Configure Transmit Parameters.vi"("Transmit Parameters"=w165, "Tx Channel"=w164) -> ("error out"=w162:errorcluster)  [unwired: 8 in, 1 out]
                  n51 = call <instrlib>:"Read MP Registry Data.vi"("error in (no error)"=w162) -> ("Micropulse Data"=w163:T41)  [unwired: 7 in, 3 out]
                  n52 = Unbundle By Name(w163) -> ("Command List"=w161:string)
                  n53 = local write "Command List"(w161) -> ()
                }
                event Value Change {
                  w167 = u32 1  # Test No.
                  n54 = event-data() -> ("NewVal"=w171:T11)  [unwired: 1 in, 5 out]
                  n55 = call <instrlib>:"Configure Receive Parameters.vi"("Receive Parameters"=w171, "Test No."=w167) -> ("error out"=w170:errorcluster)  [unwired: 7 in, 2 out]
                  n56 = call <instrlib>:"Read MP Registry Data.vi"("error in (no error)"=w170) -> ("Micropulse Data"=w168:T41)  [unwired: 7 in, 3 out]
                  n57 = Unbundle By Name(w168) -> ("Command List"=w169:string)
                  n58 = local write "Command List"(w169) -> ()
                }
                event Value Change {
                  w172 = u32 1  # Test Number
                  n59 = event-data() -> ("NewVal"=w176:T19)  [unwired: 1 in, 5 out]
                  n60 = call <instrlib>:"Configure Multi Gate Parameters.vi"("Multi Gate Inspection"=w176, "Test Number"=w172) -> ("error out"=w175:errorcluster)  [unwired: 7 in, 2 out]
                  n61 = call <instrlib>:"Read MP Registry Data.vi"("error in (no error)"=w175) -> ("Micropulse Data"=w174:T41)  [unwired: 7 in, 3 out]
                  n62 = Unbundle By Name(w174) -> ("Command List"=w173:string)
                  n63 = local write "Command List"(w173) -> ()
                }
                event Value Change {
                  w177 = u32 1  # Test Number
                  n64 = event-data() -> ()  [unwired: 1 in, 6 out]
                  n65 = local read "Echo Gate Parameters"() -> (w180:T23)
                  n66 = local read "Echo Gate Mode"() -> (w181:T24)
                  n67 = call <instrlib>:"Configure Echo Gate Parameters.vi"("Echo Gate Parameters"=w180, "Echo Trigger Mode"=w181, "Test Number"=w177) -> ("error out"=w182:errorcluster)  [unwired: 6 in, 2 out]
                  n68 = call <instrlib>:"Read MP Registry Data.vi"("error in (no error)"=w182) -> ("Micropulse Data"=w179:T41)  [unwired: 7 in, 3 out]
                  n69 = Unbundle By Name(w179) -> ("Command List"=w178:string)
                  n70 = local write "Command List"(w178) -> ()
                }
                event "Start Acquisition": Value Change {
                  n71 = event-data() -> ()  [unwired: 1 in, 6 out]
                  n72 = call <instrlib>:"Start Continuous Test Cycles [STP].vi"() -> ()  [unwired: 10 in, 2 out]
                }
                event "Stop Acquisition": Value Change {
                  w183 = TRUE  # Erase All? (def F)
                  n73 = event-data() -> ()  [unwired: 1 in, 6 out]
                  n74 = call <instrlib>:"Enter Idle Mode [STX].vi"("Erase All? (def T)"=w183) -> ()  [unwired: 9 in, 2 out]
                }
                event "Acquire Single Scan": Value Change {
                  n75 = event-data() -> ()  [unwired: 1 in, 6 out]
                  n76 = call <instrlib>:"Start 1 Test Cycle [CAL].vi"() -> ()  [unwired: 10 in, 2 out]
                }
                event "A-Scan + Peaks": Scale Range Change {
                  n77 = event-data() -> ()  [unwired: 1 in, 8 out]
                  n78 = call <instrlib>:"Force Gate Update On XY Chart.vi"("Set?"=TRUE, "Test No."=u32 1) -> ()  [unwired: 7 in, 3 out]
                }
                event Value Change {
                  w186 = TRUE
                  # "Stop all activity and reset the hardware to change the sampling frequency"
                  n79 = event-data() -> ()  [unwired: 1 in, 6 out]
                  n80 = local write "Stop"(w186) -> ()
                }
                event Value Change {
                  n81 = event-data() -> ("NewVal"=w188:T25)  [unwired: 1 in, 5 out]
                  n82 = call <instrlib>:"Set Encoder Mode [ENCM].vi"("Encoder Mode"=w188) -> ()  [unwired: 9 in, 2 out]
                }
                event Value Change {
                  n83 = event-data() -> ("NewVal"=w190:T26)  [unwired: 1 in, 5 out]
                  n84 = call <instrlib>:"Set Encoder Settings.vi"("Encoder Settings"=w190, "Axis No."="Axis No.") -> ()  [unwired: 9 in, 1 out]
                }
                event "Set Position": Value Change {
                  w191 = u8 1  # Axis No.
                  n85 = event-data() -> ()  [unwired: 1 in, 6 out]
                  n86 = call <instrlib>:"Set Encoder Position [LCP].vi"("Position (mm)"="Position To Set", "Axis No."=w191) -> ()  [unwired: 8 in, 2 out]
                }
                event Value Change {
                  n87 = event-data() -> ("NewVal"=w194:T1)  [unwired: 1 in, 5 out]
                  n88 = call <instrlib>:"MicroPulse Intensity Colour Tables.vi"("Colour Map Type"=w194) -> ("Colour Table"=w193:u32[])  [unwired: 10 in]
                  n89 = property on="B-Scan Chart" class="IntGraph (strict)"("Color Table"=w193) -> ()  [unwired: 2 in, 2 out]
                }
                event "Get Status": Value Change {
                  n90 = event-data() -> ()  [unwired: 1 in, 6 out]
                  n91 = call <instrlib>:"Get Status Info [STS].vi"("Request System Status"="Request System Status") -> ()  [unwired: 9 in, 2 out]
                }
                event "Start FLZ Test": Value Change {
                  w201 = u8 1  # Axis No.
                  # "Stop any acquisition that's going on"
                  n92 = event-data() -> ()  [unwired: 1 in, 6 out]
                  n93 = call <instrlib>:"Enter Idle Mode [STX].vi"() -> ("error out"=w203:errorcluster)  [unwired: 10 in, 1 out]
                  n94 = call <instrlib>:"Start Scan (Start to End).vi"("error in (no error)"=w203, "Scan definition"="FLZ Scan definition", "Axis No."=w201) -> ("error out"=w200:errorcluster)  [unwired: 7 in, 1 out]
                  n95 = call <instrlib>:"FGV-B-Scan Active.vi"("Action"=FGV_-_B-Scan_Active_-_Action_[Enum]."Start B-Scan", "error in (no error)"=w200) -> ("error out"=w197:errorcluster)  [unwired: 7 in, 2 out]
                  n96 = call <instrlib>:"Read MP Registry Data.vi"("error in (no error)"=w197) -> ("Micropulse Data"=w199:T41)  [unwired: 7 in, 3 out]
                  n97 = Unbundle By Name(w199) -> ("Command List"=w198:string)
                  n98 = local write "Command List"(w198) -> ()
                }
                event "Start FLR Test": Value Change {
                  w205 = u8 1  # Axis No.
                  # "Stop any acquisition that's going on"
                  n99 = event-data() -> ()  [unwired: 1 in, 6 out]
                  n100 = call <instrlib>:"Enter Idle Mode [STX].vi"() -> ("error out"=w207:errorcluster)  [unwired: 10 in, 1 out]
                  n101 = call <instrlib>:"Start Scan (Relative [FLR]).vi"("error in (no error)"=w207, "Scan definition"="FLR Scan definition", "Axis No."=w205) -> ("error out"=w206:errorcluster)  [unwired: 7 in, 1 out]
                  n102 = call <instrlib>:"FGV-B-Scan Active.vi"("Action"=FGV_-_B-Scan_Active_-_Action_[Enum]."Start B-Scan", "error in (no error)"=w206) -> ("error out"=w209:errorcluster)  [unwired: 7 in, 2 out]
                  n103 = call <instrlib>:"Read MP Registry Data.vi"("error in (no error)"=w209) -> ("Micropulse Data"=w211:T41)  [unwired: 7 in, 3 out]
                  n104 = Unbundle By Name(w211) -> ("Command List"=w210:string)
                  n105 = local write "Command List"(w210) -> ()
                }
                event "Start Timed Test": Value Change {
                  # "use property node so we can sequence starting\nthe B-Scan acitve flags and then enabling the timer"
                  # "Stop any acquisition that's going on"
                  n106 = event-data() -> ()  [unwired: 1 in, 6 out]
                  n107 = call <instrlib>:"Enter Idle Mode [STX].vi"() -> ("error out"=w214:errorcluster)  [unwired: 10 in, 1 out]
                  n108 = call <instrlib>:"FGV-B-Scan Active.vi"("Action"=FGV_-_B-Scan_Active_-_Action_[Enum]."Start B-Scan", "error in (no error)"=w214) -> ("error out"=w213:errorcluster)  [unwired: 7 in, 2 out]
                  n109 = property on="Scan Timer Enabled?" class="Bool (strict)"(error in=w213, "Value"=TRUE ("Scan Timer Enabled?")) -> ()  [unwired: 1 in, 2 out]
                }
                event Key Down {
                  n110 = event-data() -> ("Char"=w216:i16)  [unwired: 1 in, 7 out]
                  n111 = case shown="32" w216 {
                    frame 0, Default {
                    }
                    frame 32 {
                      # "Space bar - Stops all scan activity - returns micropulse to idle mode"
                      n112 = call <instrlib>:"FGV-B-Scan Active.vi"() -> ("B-Scan In Progress?"=w217:bool)  [unwired: 9 in, 2 out]
                      n113 = case shown="True" w217 {
                        frame False {
                        }
                        frame True {
                          n114 = call <instrlib>:"Enter Idle Mode [STX].vi"() -> ("error out"=w218:errorcluster)  [unwired: 10 in, 1 out]
                          n115 = call <instrlib>:"FGV-B-Scan Active.vi"("Action"=FGV_-_B-Scan_Active_-_Action_[Enum]."B-Scan Finished", "error in (no error)"=w218) -> ()  [unwired: 7 in, 3 out]
                        }
                      }
                    }
                  }
                }
                event "Stop Test": Value Change {
                  # "Stops all scan activity - returns micropulse to idle mode\nHitting the Spacebar also does this."
                  n116 = event-data() -> ()  [unwired: 1 in, 5 out]
                  n117 = call <instrlib>:"FGV-B-Scan Active.vi"() -> ("B-Scan In Progress?"=w220:bool)  [unwired: 9 in, 2 out]
                  n118 = case shown="True" w220 {
                    frame False {
                    }
                    frame True {
                      n119 = call <instrlib>:"Enter Idle Mode [STX].vi"() -> ("error out"=w221:errorcluster)  [unwired: 10 in, 1 out]
                      n120 = call <instrlib>:"FGV-B-Scan Active.vi"("Action"=FGV_-_B-Scan_Active_-_Action_[Enum]."B-Scan Finished", "error in (no error)"=w221) -> ()  [unwired: 7 in, 3 out]
                    }
                  }
                }
                event "Centre Cursor": Value Change {
                  n121 = event-data() -> ()  [unwired: 1 in, 6 out]
                  n122 = property on="B-Scan Chart" class="IntGraph (strict)"() -> ("XScale.Maximum"=w228:dbl, "XScale.Minimum"=w224:dbl)  [unwired: 2 in, 2 out]
                  n123 = Subtract(x=w228, y=w224) -> (x-y=w227:dbl)
                  n124 = Divide(x=w227, y=2.0) -> (x/y=w225:dbl)
                  n125 = Add(x=w225, y=w224) -> (x+y=w223:dbl)
                  n126 = property on="B-Scan Chart" class="IntGraph (strict)"("Cursor.Cursor X"=w223) -> ()  [unwired: 2 in, 2 out]
                }
                event "B-Scan Chart": Cursor Move {
                  n127 = event-data() -> ()  [unwired: 1 in, 8 out]
                  n128 = property on="B-Scan Chart" class="IntGraph (strict)"() -> ("Cursor.Cursor Position"=w229:T46, "Value"=w237:u16[][])  [unwired: 2 in, 2 out]
                  n129 = Unbundle By Name(w229) -> ("Cursor X"=w236:dbl)
                  n130 = property on="A-Scan + Peaks" class="XYGraph (strict)"() -> ("XScale.Multiplier"=w235:dbl, "XScale.Offset"=w234:dbl)  [unwired: 2 in, 2 out]
                  n131 = Index Array(array=w237, index (row)=w236) -> (element=w232:u16[])  [unwired: 1 in]
                  n132 = for {
                    tunnel: w232 -> [_] mode=indexing
                    tunnel: w235 -> [w242]
                    tunnel: w234 -> [w239]
                    tunnel: [w238] -> w233 mode=indexing
                    i -> [w241]
                    n133 = Multiply(x=w242, y=w241) -> (x*y=w240:dbl)
                    n134 = Subtract(x=w240, y=w239) -> (x-y=w238:dbl)
                  }
                  n135 = Bundle(w233, "Value"=w232) -> (w231:cluster{dbl[], "Value":u16[]})  [unwired: 1 in]
                  n136 = Build Array(w231) -> (w230:cluster{dbl[], "Value":u16[]}[])
                  n137 = local write "A-Scan + Peaks"(w230) -> ()
                }
                event Panel Close? {
                  n138 = event-data() -> ()  [unwired: 1 in, 4 out]
                  n139 = event-data("Discard?"=TRUE) -> ()  [unwired: 1 in, 1 out]
                }
                event "QUIT": Value Change {
                  # "set flag to stop acquisition loop"
                  n140 = event-data() -> ()  [unwired: 1 in, 6 out]
                  n141 = call <instrlib>:"FGV-B-Scan Active.vi"("Action"=FGV_-_B-Scan_Active_-_Action_[Enum]."B-Scan Finished") -> ("B-Scan In Progress?"=w245:bool)  [unwired: 8 in, 2 out]
                  n142 = local write "B-Scan In Progress?"(w245) -> ()
                  "Stop" <- TRUE ("Stop")
                }
              }
            }
            n143 = while {
              stop <- w68 stop-if-true
              # "Timed scan trigger loop\n(Simple for example code purposes)"
              n144 = local read "Scan Timer Enabled?"() -> (w69:bool)
              n145 = case shown="True" w69 {
                frame False {
                  # "Add a wait so the loop doesn't hog the processor"
                  n146 = Wait (ms)(milliseconds to wait=u32 100) -> ()  [unwired: 1 out]
                }
                frame True {
                  n147 = call <instrlib>:"FGV-B-Scan Active.vi"("Action"=FGV_-_B-Scan_Active_-_Action_[Enum]."Read") -> ("error out"=w72:errorcluster, "B-Scan In Progress?"=w73:bool)  [unwired: 8 in, 1 out]
                  n148 = case shown="True" w73 {
                    tunnel: w72 -> [_ w76]
                    frame False {
                      # "Reset the scan timer flag when B-Scan finishes"
                      n149 = local write "Scan Timer Enabled?"(FALSE ("Scan Timer Enabled?")) -> ()
                    }
                    frame True {
                      # "trigger a CAL 0 when time elapsed"
                      n150 = Unbundle By Name("Timed Scan definition") -> ("Update Rate"=w78:i32)
                      n151 = Wait (ms)(milliseconds to wait=w78) -> (millisecond timer value=w77:u32)
                      n152 = flat-sequence {
                        tunnel: w77 -> [_]
                        tunnel: w76 -> [w80]
                        frame #0 {
                          n153 = call <instrlib>:"Start 1 Test Cycle [CAL].vi"("error in (no error)"=w80) -> ()  [unwired: 9 in, 2 out]
                        }
                      }
                    }
                  }
                }
              }
              n154 = flat-sequence {
                tunnel: [w70] -> w68
                frame #0 {
                  n155 = local read "Stop"() -> (w70:bool)
                }
              }
            }
            n156 = control-ref of="A-Scan + Peaks"() -> (w67:refnum<vi>)
            n157 = property on="B-Scan Chart" class="IntGraph (strict)"() -> ("Plot Area Size"=w65:T47)  [unwired: 2 in, 2 out]
            n158 = while {
              tunnel: w67 -> [w85]
              tunnel: [w84] -> w64
              tunnel: w65 -> [w82]
              tunnel: [w81] -> _
              stop <- w83 stop-if-true
              # "Asynchronous Read from Micropulse"
              n159 = call <instrlib>:"Read MP Message.vi"() -> ("error out"=w86:errorcluster, "scan data info"=w87:T48, "Instrument Message"=w90:string)  [unwired: 7 in, 2 out]
              n160 = call <instrlib>:"Instrument Message History.vi"("Instrument Message"=w90) -> ("Message Count"=→"message count":i32, "Message History out"=→"System Messages":string)  [unwired: 9 in]
              n161 = Unbundle By Name(w87) -> ("Test No."=w88:u32)
              n162 = case shown="1" w88 {
                selector: w88 -> [_ w105]
                tunnel: w87 -> [_ w102]
                tunnel: w86 -> [w93 w107]
                tunnel: w85 -> [_ w104]
                tunnel: [w93 w106] -> w84
                tunnel: w82 -> [_ w95]
                tunnel: [_ w94] -> w81
                frame -1, Default {
                }
                frame 1 {
                  # "To save CPU time and allow for updates due to cursor moves, we restrict unnecessary updates from the uPulse to live data."
                  n163 = local read "Axis No."() -> (w100:u8)
                  n164 = call <instrlib>:"AScan+Peaks to XY Chart.vi"("error in (no error)"=w107, "scan data info"=w102, "Test No."=w105) -> ("error out"=w108:errorcluster, "Echo Range (us)"=w103:dbl, "AScan+Peaks"=w111:cluster{"timebase":dbl[], "data":u16[]}[], "Update Indicators?"=w98:bool, "Running Average PRF"=→"running average PRF":dbl)  [unwired: 3 in, 1 out]
                  n165 = case shown="\"Absolute Scan [FLX+FLZ]\", Default" "Scan Choice" {
                    tunnel: w102 -> [w130 w135 w141]
                    tunnel: [w124 w131 w138] -> w94
                    tunnel: [w128 w137 w142] -> w97
                    tunnel: [w127 w134 w143] -> _
                    tunnel: w100 -> [w126 w133 _]
                    tunnel: [w125 w132 w139] -> w96
                    frame "Absolute Scan [FLX+FLZ]", Default {
                      n166 = local read "FLZ Scan definition"() -> (w129:T29)
                      n167 = call <instrlib>:"B-Scan (LLC messages).vi"("Scan definition"=w129, "Axis No."=w126, "scan data info"=w130) -> ("Update Display?"=w125:bool, "B-Scan In Progress?"=w128:bool, "B-Scan index"=w127:i32, "B-Scan Out"=w124:u16[][])  [unwired: 5 in]
                    }
                    frame "Relative Scan [FLR] " {
                      n168 = local read "FLR Scan definition"() -> (w136:T31)
                      n169 = call <instrlib>:"B-Scan (Relative [FLR]).vi"("Scan definition"=w136, "Axis No."=w133, "scan data info"=w135) -> ("Update Display?"=w132:bool, "B-Scan In Progress?"=w137:bool, "B-Scan index"=w134:i32, "B-Scan Out"=w131:u16[][])  [unwired: 5 in]
                    }
                    frame "Timed Scan" {
                      n170 = local read "Timed Scan definition"() -> (w140:T33)
                      n171 = call <instrlib>:"B-Scan (Timed).vi"("Scan definition"=w140, "scan data info"=w141) -> ("Update Display?"=w139:bool, "B-Scan In Progress?"=w142:bool, "B-Scan Index"=w143:i32, "B-Scan Out"=w138:u16[][])  [unwired: 6 in]
                    }
                  }
                  "B-Scan In Progress?" <- w97
                  n172 = Index Array(array=w111, index="Gate No.") -> (element=→"peak data":cluster{"timebase":dbl[], "data":u16[]})
                  n173 = case shown="True" w98 {
                    tunnel: w111 -> [_ w119]
                    tunnel: w108 -> [w112 w117]
                    tunnel: [w112 w116] -> w106
                    tunnel: w105 -> [_ w115]
                    tunnel: w104 -> [_ w114]
                    tunnel: w103 -> [_ w113]
                    frame False {
                    }
                    frame True {
                      n174 = call <instrlib>:"Adjust Peak Offsets On XY Chart.vi"("error in (no error)"=w117, "Echo Range in"=w113, "AScan+Peaks in"=w119) -> ("error out"=w118:errorcluster, "AScan+Peaks out"=→"A-Scan + Peaks":cluster{"timebase":dbl[], "data":u16[]}[])  [unwired: 7 in]
                      n175 = call <instrlib>:"Draw Gates On XY Chart.vi"("error in (no error)"=w118, "Echo Range"=w113, "XYGraph in"=w114, "Test No."=w115) -> ("error out"=w116:errorcluster)  [unwired: 7 in]
                    }
                  }
                  "live error out" <- w106
                  n176 = case shown="True" w96 {
                    tunnel: w94 -> [_ w121]
                    tunnel: w95 -> [_ w122]
                    frame False {
                    }
                    frame True {
                      n177 = call <instrlib>:"Decimate Data For 2D Intensity Chart.vi"("Plot Area"=w122, "2D Display in"=w121) -> ("Decimated Display"=→"B-Scan Chart":u16[][])  [unwired: 9 in]
                    }
                  }
                }
              }
              n178 = flat-sequence {
                tunnel: [w92] -> w83
                tunnel: w84 -> [_]
                frame #0 {
                  n179 = local read "Stop"() -> (w92:bool)
                }
              }
            }
          }
          frame Error {
          }
        }
        n180 = Select(t=Main_Program_State_-_Enum."Reset HW", s=w59, f=Main_Program_State_-_Enum."Shutdown") -> (s? t:f=w58:T38)
      }
      frame "Reset HW" {
        # "Close the connection to allow for reopening in the \"Init HW\" case"
        n181 = call <instrlib>:"Close.vi"("error in (no error)"=w252) -> ("error out"=w251:errorcluster)  [unwired: 9 in, 1 out]
      }
      frame "Shutdown" {
        # "Terminate the TCP/IP connection"
        n182 = local write "Stop"(FALSE ("stop")) -> ()
        n183 = call <instrlib>:"Close.vi"() -> ()  [unwired: 10 in, 2 out]
      }
    }
  }
